vi "solar_voy Write (TCP).vi"(5 "TARGET":string, 6 "Suppress Errors? (T)":bool=TRUE, 7 "CMD":enum8{"CMD", "TLM"}(ring), 8 "error in (no error)":errorcluster, 10 "TCP Data to Send":string, 11 "Voyager Refnum in":T1) -> (0 "error out":errorcluster, 2 "TCP Data Sent":string, 3 "Voyager Refnum out":T1)   [LabVIEW 2018]
doc: "This writes the raw TCP message. The TCP Data must contain the header item. The 'HDR_LENGTH' item gets updated before the TCP data is sent."
uses:
  solar_voy_ctl Voyager Refnum.ctl
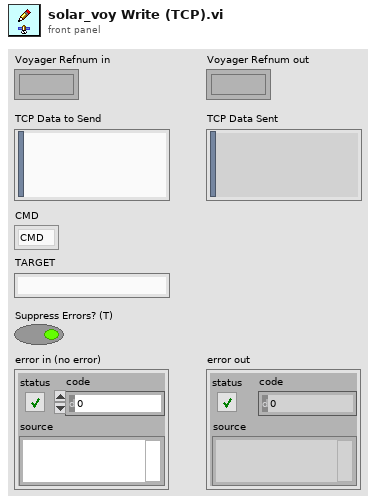
[diagram p1: front panel]
types:
  T1 = typedef "solar_voy_ctl Voyager Refnum.ctl" = refnum<k1>
  T2 = typedef "solar_voy_ctl Voyager.ctl" = cluster{"PACKETS":T3[], "COSMOS_Root":path, "CMD_HDR":T8, "TLM_HDR":T8, "TCPs":T9[], "VoyagerIDOffset":cluster{"VoyagerIDOffset":u16[], "Target Names":string[]}}
  T3 = typedef "solar_voy_def_ctl PACKET.ctl" = cluster{"PACKET_ID":T4, "ENDIAN":enum8{"BIG", "LITTLE"}, "DESC":string, "HZRD":bool, "ITEMS":T5[], "NoExport":bool, "last_time":timestamp, "last_count":u32, "last_data":string}
  T4 = typedef "solar_voy_def_ctl PACKET_ID.ctl" = cluster{"ID":u16, "CMD":enum8{"CMD", "TLM"}, "TARGET":string, "PACKET":string}
  T5 = typedef "solar_voy_def_ctl ITEM.ctl" = cluster{"NAME":string, "OFFSET":i32, "SIZE":i32, "TYPE":T6, "EACH_SIZE":i32, "LVTYPE":T7, "MIN":dbl, "MAX":dbl, "DEFAULT":string, "DESC":string, "ID":bool, "MODIFIERS":variant, "last_value":variant}
  T6 = typedef "solar_voy_def_ctl ITEM TYPE.ctl" = enum8{"BLOCK", "INT", "UINT", "FLOAT", "STRING"}
  T7 = typedef "solar_type Item Type.ctl" = enum16{"NULL", "UNKNOWN", "CLUSTER", "I8", "I16", "I32", "I64", "U8", "U16", "U32", "U64", "U8_ENUM", "U16_ENUM", "U32_ENUM", "SGL", "DBL", "BOOLEAN", "STRING", "PATH", "VISA", "TAG", "TIME", "I8_1D", "I16_1D", "I32_1D", "I64_1D", "U8_1D", "U16_1D", "U32_1D", "U64_1D", "U8_ENUM_1D", "U16_ENUM_1D", "U32_ENUM_1D", "SGL_1D", "DBL_1D", "BOOLEAN_1D", "STRING_1D", "PATH_1D", "VISA_1D", "TAG_1D", "TIME_1D", "I8_2D", "I16_2D", "I32_2D", "I64_2D", "U8_2D", "U16_2D", "U32_2D", "U64_2D", "U8_ENUM_2D", "U16_ENUM_2D", "U32_ENUM_2D", "SGL_2D", "DBL_2D", "BOOLEAN_2D", "STRING_2D", "PATH_2D", "VISA_2D", "TAG_2D", "TIME_2D"}
  T8 = typedef "solar_voy_def_ctl HDR.ctl" = cluster{"ITEMS":T5[], "LENGTH_NAME":string, "LENGTH_VALUE_OFFSET":i32, "ID_NAME":string, "ENDIAN":enum8{"BIG", "LITTLE"}, "GUID_NAME":string, "DEFAULT_TARGET":string, "DEFAULT_PACKET":string, "DEFAULT_ERROR":string}
  T9 = typedef "solar_voy_ctl TCP.ctl" = cluster{"Connected":bool, "Port":u16, "Listener":refnum<k5>, "ServerIP":string, "TCP":refnum<k5>, "Setup":T10, "VIRefnum":refnum<vi>, "TARGETS_CMD":string[], "TARGETS_TLM":string[]}
  T10 = typedef "solar_voy_ctl Port Setup.ctl" = enum8{"SERVER", "CLIENT", "SERVER_CMD", "SERVER_TLM"}
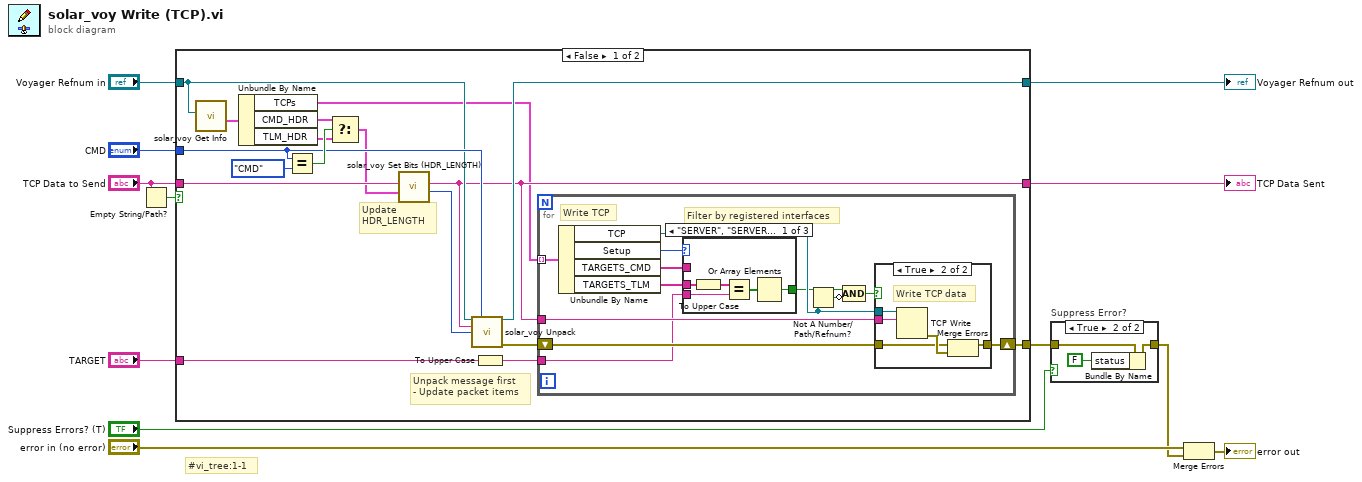
[diagram p0: block diagram]
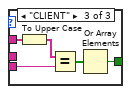
[diagram p3: hidden frame]
diagram:
  # "#vi_tree:1-1"
  n1 = Empty String/Path?(string/path="TCP Data to Send") -> (empty?=w2:bool)
  n2 = case shown="False" w2 {
    tunnel: "TCP Data to Send" -> [w21 _]
    tunnel: [w17 _] -> w8
    tunnel: "CMD" -> [w24 _]
    tunnel: [w14 _] -> w6
    tunnel: "Voyager Refnum in" -> [w23 w58]
    tunnel: [w22 w58] -> w4
    tunnel: "TARGET" -> [w18 _]
    frame False {
      # "Update\nHDR_LENGTH"
      # "Unpack message first\n- Update packet items"
      n3 = call "solar_voy Get Info.vi"("Voyager Refnum"=w23) -> ("Voyager"=w29:T2)  [unwired: 8 in, 2 out]
      n4 = Unbundle By Name(w29) -> ("TCPs"=w13:T9[], "CMD_HDR"=w26:T8, "TLM_HDR"=w25:T8)
      n5 = Equal?(x=w24, y=enum8{"CMD", "TLM"}."CMD") -> (x = y?=w27:bool)
      n6 = Select(t=w26, s=w27, f=w25) -> (s? t:f=w19:T8)
      n7 = call "solar_voy Set Bits (HDR_LENGTH).vi"("HDR"=w19, "TCP Data (No HDR_LENGTH)"=w21) -> ("HDR_ID"=w20:u16, "TCP Data out"=w14:string)  [unwired: 8 in]
      n8 = call "solar_voy Unpack.vi"("Voyager Refnum in"=w23, "CMD"=w24, "TCP Data"=w14, "ID"=w20) -> ("Voyager Refnum out"=w22:T1, "error out"=w15:errorcluster)  [unwired: 5 in, 5 out]
      n9 = To Upper Case(1:w18) -> (0:w16:string)
      n10 = for {
        tunnel: w13 -> [w41] mode=indexing
        tunnel: w14 -> [w39]
        shift-right: [w37] -> w17
        shift-left: w15 -> [w38]
        tunnel: w16 -> [w35]
        # "Filter by registered interfaces"
        # "Write TCP"
        n11 = Unbundle By Name(w41) -> ("TCP"=w40:refnum<k5>, "Setup"=w34:T10, "TARGETS_CMD"=w33:string[], "TARGETS_TLM"=w36:string[])
        n12 = case shown="\"SERVER\", \"SERVER_TLM\"" w34 {
          tunnel: w36 -> [w46 _ _]
          tunnel: w35 -> [w45 _ w51]
          tunnel: w33 -> [_ _ w47]
          tunnel: [w42 _ w48] -> w30
          frame "SERVER", "SERVER_TLM" {
            n13 = To Upper Case(1:w46) -> (0:w44:string[])
            n14 = Equal?(x=w44, y=w45) -> (x = y?=w43:bool[])
            n15 = Or Array Elements(Boolean array=w43) -> (logical OR=w42:bool)
          }
          frame "SERVER_CMD" {
            # "Do not \nsend TLM"
          }
          frame "CLIENT" {
            n16 = To Upper Case(1:w47) -> (0:w50:string[])
            n17 = Equal?(x=w50, y=w51) -> (x = y?=w49:bool[])
            n18 = Or Array Elements(Boolean array=w49) -> (logical OR=w48:bool)
          }
        }
        n19 = Not A Number/Path/Refnum?(number/path/refnum=w40) -> (NaN/Path/Refnum?=w32:bool)
        n20 = Compound Arithmetic op=AND(w30, invert w32) -> (w31:bool)
        n21 = case shown="True" w31 {
          tunnel: w40 -> [_ w57]
          tunnel: w39 -> [_ w56]
          tunnel: w38 -> [w52 w54]
          tunnel: [w52 w53] -> w37
          frame False {
          }
          frame True {
            # "Write TCP data"
            n22 = TCP Write(connection ID=w57, data in=w56) -> (error out=w55:errorcluster)  [unwired: 1 in, 3 out]
            n23 = Merge Errors(w54, w55) -> (w53:errorcluster)
          }
        }
      }
    }
    frame True {
      # "Invalid Message to Send\n- Do nothing"
    }
  }
  "Voyager Refnum out" <- w4
  "TCP Data Sent" <- w6
  n24 = case "Suppress Error?" shown="True" "Suppress Errors? (T)" {
    tunnel: w8 -> [w59 w62]
    tunnel: [w59 w61] -> w10
    frame False {
    }
    frame True {
      n25 = Bundle By Name(cluster=w62, "status"=FALSE) -> (w61:errorcluster)
    }
  }
  n26 = Merge Errors("error in (no error)", w10) -> (→"error out":errorcluster)
